vi "Drive.vi"(8 "error in":errorcluster, 10 "RobotPosition":cluster{"X":dbl, "Y":dbl, "Angle":dbl}, 11 "Movements":cluster{"Left":dbl, "Right":dbl}[](array[cluster])) -> (0 "error out":errorcluster, 1 "deltaPosition":cluster{"X":dbl, "Y":dbl, "Angle":dbl}, 2 "state out":T1)   [LabVIEW 2009, in "Main.lvlib"]
doc: "Main drive algorithm of the robot. Calculates robot's movement to reach specified in Relative Coordinates point, then drives robot according to calculated movements. Also updates state of the robot based on information from the controllers. Enables or disables collision avoidance algorithm depending on the movement type."
uses:
  Main.lvlib
  MainVariables.lvlib
  Drive.lvlib
  Drive/Drive_Utils.lvlib
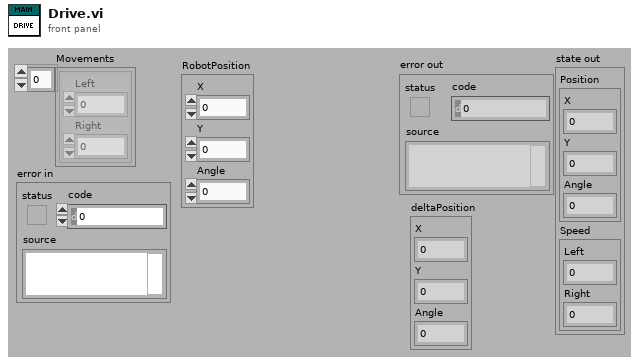
[diagram p1: front panel]
types:
  T1 = cluster{"Position":cluster{"X":dbl, "Y":dbl, "Angle":dbl}, "Speed":cluster{"Left":dbl, "Right":dbl}}
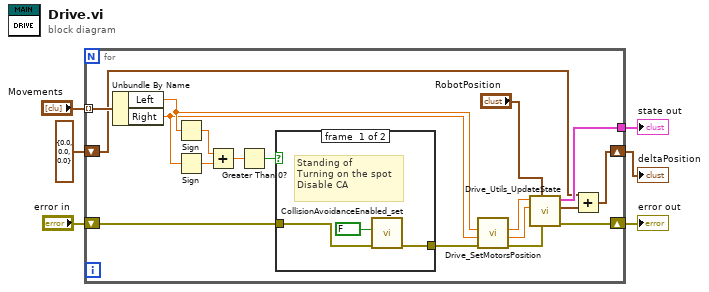
[diagram p0: block diagram]
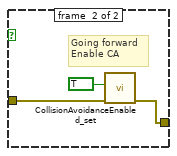
[diagram p2: hidden frame]
diagram:
  n1 = for {
    tunnel: "Movements" -> [w24] mode=indexing
    shift-right: [w14] -> w6
    shift-left: "error in" -> [w19]
    tunnel: [w11] -> w5
    shift-right: [w9] -> w1
    shift-left: cluster{"X":dbl, "Y":dbl, "Angle":dbl} {"X"=0.0, "Y"=0.0, "Angle"=0.0} -> [w8]
    n2 = Unbundle By Name(w24) -> ("Left"=w17:dbl, "Right"=w16:dbl)
    n3 = Sign(1:w17) -> (0:w23:dbl)
    n4 = Sign(1:w16) -> (0:w22:dbl)
    n5 = Add(x=w23, y=w22) -> (x+y=w21:dbl)
    n6 = Greater Than 0?(x=w21) -> (x > 0?=w20:bool)
    n7 = case shown="True" w20 {
      tunnel: w19 -> [w26 w30]
      tunnel: [w25 w29] -> w18
      frame #0 {
        # "Standing of\nTurning on the spot\nDisable CA"
        n8 = call "CollisionAvoidanceEnabled_set.vi"("error in (no error)"=w26, "Enabled? (T)"=FALSE) -> ("error out"=w25:errorcluster)  [unwired: 9 in]
      }
      frame #1 {
        # "Going forward\nEnable CA"
        n9 = call "CollisionAvoidanceEnabled_set.vi"("error in (no error)"=w30, "Enabled? (T)"=TRUE) -> ("error out"=w29:errorcluster)  [unwired: 9 in]
      }
    }
    n10 = call "Drive_SetMotorsPosition.vi"("error in (no error)"=w18, "Distance Right"=w16, "Distance Left"=w17) -> ("error out"=w15:errorcluster, "Distance Right out"=w12:dbl, "Distance Left out"=w13:dbl)  [unwired: 6 in]
    n11 = call "Drive_Utils_UpdateState.vi"("error in (no error)"=w15, "RobotPosition"="RobotPosition", "delta right"=w12, "delta left"=w13) -> ("error out"=w14:errorcluster, "deltaPosition"=w10:cluster{"X":dbl, "Y":dbl, "Angle":dbl}, "state out"=w11:T1)  [unwired: 5 in]
    n12 = Add(x=w8, y=w10) -> (x+y=w9:cluster{"X":dbl, "Y":dbl, "Angle":dbl})
  }
  "error out" <- w6
  "state out" <- w5
  "deltaPosition" <- w1
